vi "FTW-Ether-Construct.vi"(5 "FTW Ether Configuration":T1="{\n  \"ApplicationName\": \"Featherweight Application\",\n  \"ApplicationVersion\": \"0.1.0-1\"\n}", 11 "error in":errorcluster) -> (15 "error out":errorcluster)   [LabVIEW 2012, in "FTW-Actor.lvlib" / "FTW-Ether.lvclass"]
uses:
  FTW-Ether.lvclass
  Utility/FTW-Actor-Configuration.ctl
  <instcachedir>/0/FTW-JSON-ToLabVIEW_0E3E72F634BF4A9AB33E22111E055A26.lvgen/FTW-JSON-ToLabVIEW_0E3E72F634BF4A9AB33E22111E055A26_001.vi
  Core/JSON/FTW-JSON-RegexParse.vi
  Core/Regex/FTW-Regex.vi
  FTW-Ether-Instance.vi
  Core/JSON/FTW-JSON-RegexHeader.vi
  Core/Error/FTW-ERR-ThrowError.vi
  Core/Error/FTW-ERR-ThrowGenericError.vi
  Core/Container/FTW-Container-Construct.vi
  Core/Container/FTW-Container-Load-JSON.vi
  Core/Container/FTW-Container-Destroy.vi
  EventLogger/FTW-Logger.lvclass
  ZMQ/FTW-Endpoint-ZMQ.lvclass
  Utility/FTW-Actor-Address.ctl
  FTW-Actor.lvlib
panel:
  # "Inputs"
  # "Outputs"
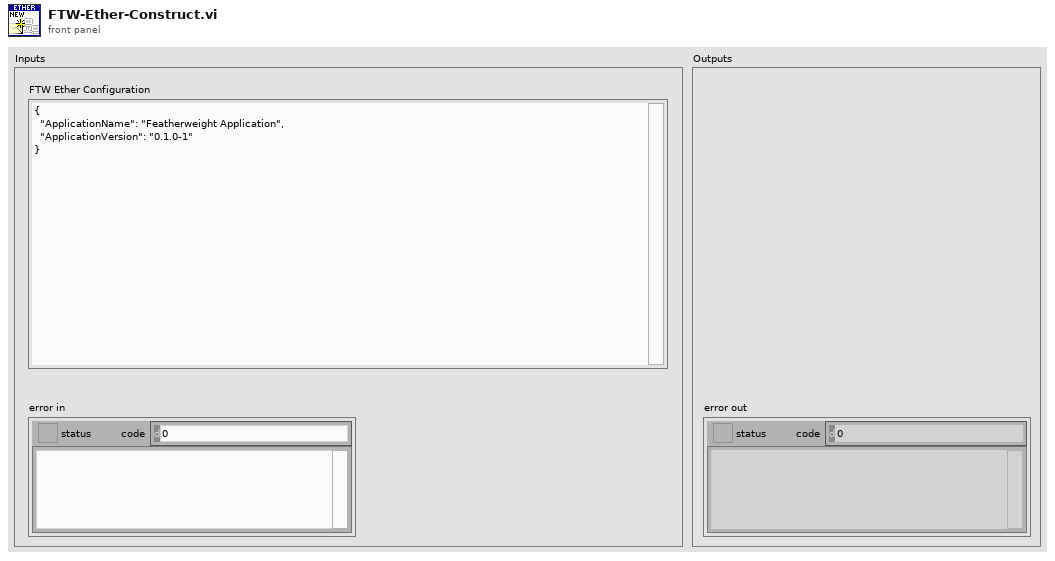
[diagram p1: front panel]
types:
  T1 = typedef "FTW-Actor.lvlib/FTW-Actor-Configuration.ctl" = string
  T2 = typedef "FTW-Actor.lvlib/FTW-Actor-Address.ctl" = string
  T3 = cluster{"ApplicationName":string, "ApplicationVersion":string, "LoggerAddress":T2, "LoggerDirectory":string, "LoggerDiskThrashDelay":u32}
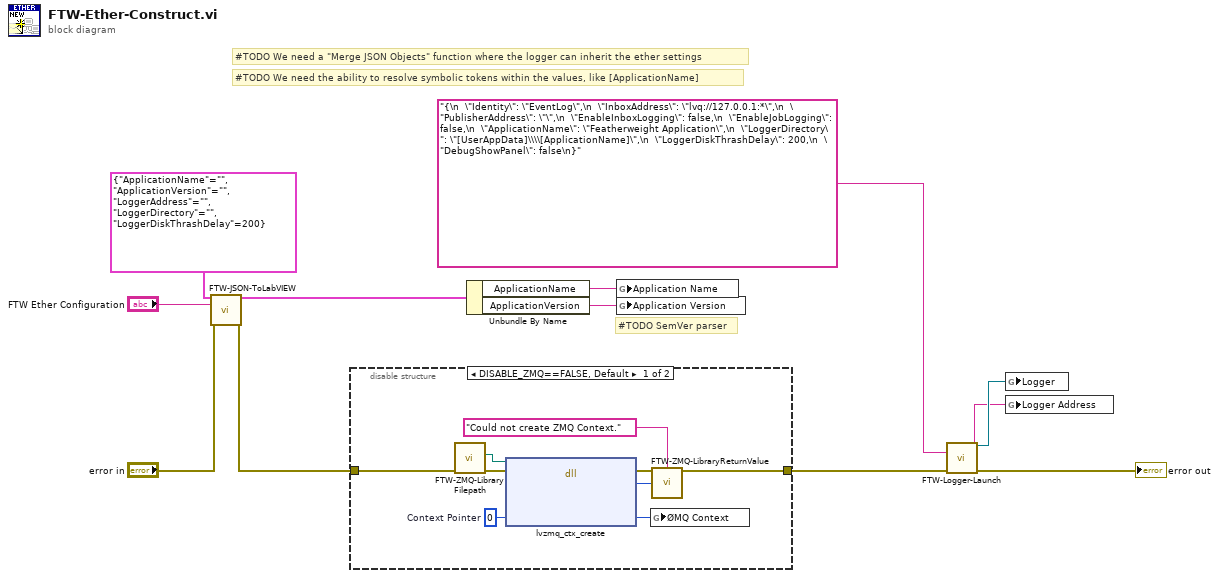
[diagram p0: block diagram]
diagram:
  # "#TODO SemVer parser"
  # "#TODO We need the ability to resolve symbolic tokens within the values, like [ApplicationName]"
  # "#TODO We need a \"Merge JSON Objects\" function where the logger can inherit the ether settings"
  n1 = call-generic "FTW-JSON-ToLabVIEW.vi"("Type and Defaults"=T3 {"ApplicationName"="", "ApplicationVersion"="", "LoggerAddress"="", "LoggerDirectory"="", "LoggerDiskThrashDelay"=200}, "JSON String"="FTW Ether Configuration", "error in"="error in") -> ("Populated Values"=w10:T3, "error out"=w6:errorcluster)  [unwired: 11 in]
  n2 = disable-structure shown="DISABLE_ZMQ==FALSE, Default" {
    disable-tunnel: w6 -> [w21 w22]
    disable-tunnel: [w20 w22] -> w12
    frame condition #0 (active) {
      w13 = u64 0  # Context Pointer
      n3 = call "FTW-ZMQ-LibraryFilepath.vi"("error in"=w21) -> ("error out"=w19:errorcluster, "FTW-ZMQ Library Filepath"=w16:path)  [unwired: 8 in, 1 out]
      n4 = dll-call lib="?" fn="lvzmq_ctx_create" ("zmq_labview.dll:lvzmq_init")(path in=w16, error in=w19, "Context Pointer"=w13) -> (error out=w18:errorcluster, "Return Value"=w17:i32, "Context Pointer"=w14:u64)  [unwired: 3 in, 1 out]
      n5 = global write "FTW-Ether-Instance.vi" "ØMQ Context"(w14) -> ()
      n6 = call "FTW-ZMQ-LibraryReturnValue.vi"("error in"=w18, "Error Message"="Could not create ZMQ Context.", "Return Value"=w17) -> ("error out"=w20:errorcluster)  [unwired: 12 in]
    }
    frame condition #1 {
      # "No construction is necessary if only LabVIEW\nmessage transport mechanisms are going to\nbe used."
    }
  }
  n7 = Unbundle By Name(w10) -> ("ApplicationName"=w9:string, "ApplicationVersion"=w4:string)
  n8 = global write "FTW-Ether-Instance.vi" "Application Name"(w9) -> ()
  n9 = global write "FTW-Ether-Instance.vi" "Application Version"(w4) -> ()
  n10 = call "FTW-Logger-Launch.vi"("FTW Logger Configuration"=T1 "{\n  \"Identity\": \"EventLog\",\n  \"InboxAddress\": \"lvq://127.0.0.1:*\",\n  \"PublisherAddress\": \"\",\n  \"EnableInboxLogging\": false,\n  \"EnableJobLogging\": false,\n  \"ApplicationName\": \"Featherweight Application\",\n  \"LoggerDirectory\": \"[UserAppData]\\\\[ApplicationName]\",\n  \"LoggerDiskThrashDelay\": 200,\n  \"DebugShowPanel\": false\n}" ("Logger Configuration"), "error in"=w12) -> ("FTW Logger Connector"=w3:refnum<class "FTW-Logger.lvclass">, "Logger Address"=w2:T2, "error out"=→"error out":errorcluster)  [unwired: 11 in]
  n11 = global write "FTW-Ether-Instance.vi" "Logger"(w3) -> ()
  n12 = global write "FTW-Ether-Instance.vi" "Logger Address"(w2) -> ()
